vi "Validate.vi"(7 "PwdMgr in":refnum<class "PwdMgr.lvclass">, 8 "error in (no error)":errorcluster, 11 "Userinfo":T1={"UserName"="", "Password"="", "Role"=enum."Admin"}) -> (0 "error out":errorcluster, 2 "Valid?":bool, 3 "Userinfo out":T1={"UserName"="", "Password"="", "Role"=enum."Admin"})   [LabVIEW 2020, in "Login-UI.lvlib" / "PwdMgr.lvclass"]
uses:
  PwdMgr.lvclass
  _Typedef/User-Info.ctl
  _Typedef/User-Role.ctl
  _support/_password_db_oper.ctl
  Login-UI.lvlib
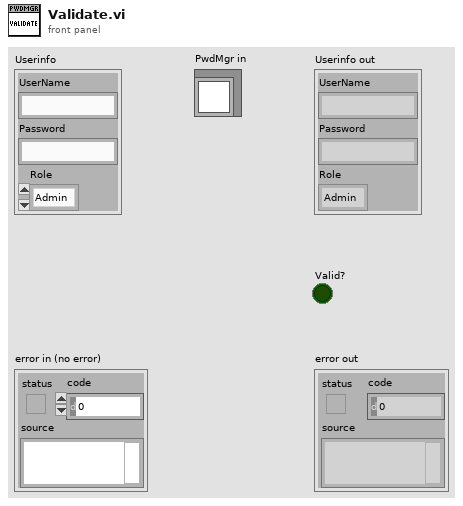
[diagram p1: front panel]
types:
  T1 = typedef "Login-UI.lvlib/User-Info.ctl" = cluster{"UserName":string, "Password":string, "Role":T2}
  T2 = typedef "Login-UI.lvlib/User-Role.ctl" = enum16{"INVALID", "Operator", "Engineer", "Admin", "Anonymous"}
  T3 = typedef "Login-UI.lvlib/PwdMgr.lvclass/_password_db_oper.ctl" = enum16{"Validate", "Register", "Unregister", "View"}
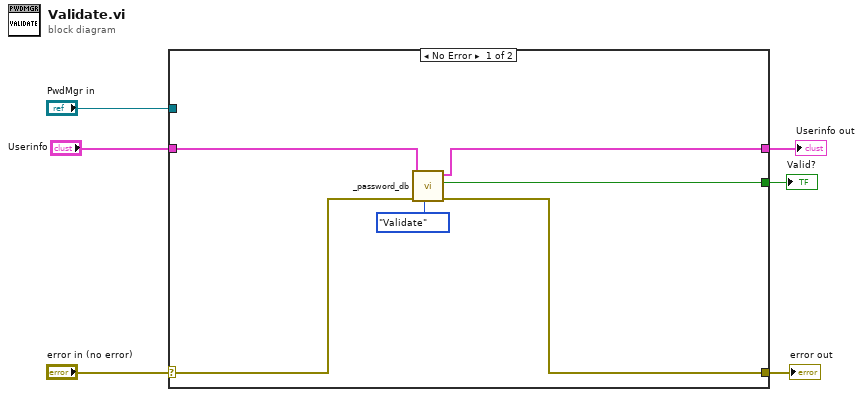
[diagram p0: block diagram]
diagram:
  n1 = case shown="No Error" "error in (no error)" {
    selector: "error in (no error)" -> [w10 w14]
    tunnel: [w9 w14] -> w5
    tunnel: "PwdMgr in" -> [_ _]
    tunnel: "Userinfo" -> [w11 w13]
    tunnel: [w8 _] -> w2
    tunnel: [w7 w13] -> w1
    frame No Error {
      n2 = call "_password_db.vi"("Enum"=_password_db_oper."Validate", "Error in"=w10, "Userinfo"=w11) -> ("Error out"=w9:errorcluster, "Boolean"=w8:bool, "Userinfo (dup)"=w7:T1)  [unwired: 5 in, 1 out]
    }
    frame Error {
    }
  }
  "error out" <- w5
  "Valid?" <- w2
  "Userinfo out" <- w1
